vi "2020.1.04生产者消费者地图调用——主vi.vi"() -> ()   [LabVIEW 2018]
uses:
  <vilib>/Instr/_visa.llb/VISA Configure Serial Port (Instr).vi
panel:
  in  "毫秒倍数":u16
  in  "滑动杆":u8(slide) scale=10.0..19.0
  out "十进制合成纬度":dbl format="%#.6g"
  out "十进制合成经度":dbl format="%#.6g"
  out "纬分":dbl
  out "纬度":i32
  out "经分":dbl
  out "经度":i32
  in  "parity (0:none)":enum16{"None", "Odd", "Even", "Mark", "Space"}(ring) caption="奇偶（0:无）"
  in  "data bits (8)":u16=8 caption="数据比特(8)" min=5 max=8 step=1
  in  "baud rate (9600)":u32=9600 caption="波特率(9600)"
  in  "VISA resource name":refnum<visa-resource-name> caption="VISA资源名称"
  in  "WebBrowser":refnum<k7>(container) caption="网页浏览器"
  in  "stop":bool caption="停止"
  out "读取缓冲区":string
  out "定位是否成功":bool
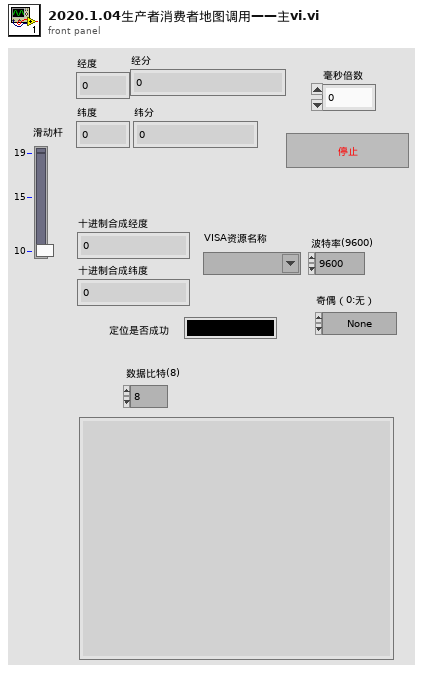
[diagram p1: front panel]
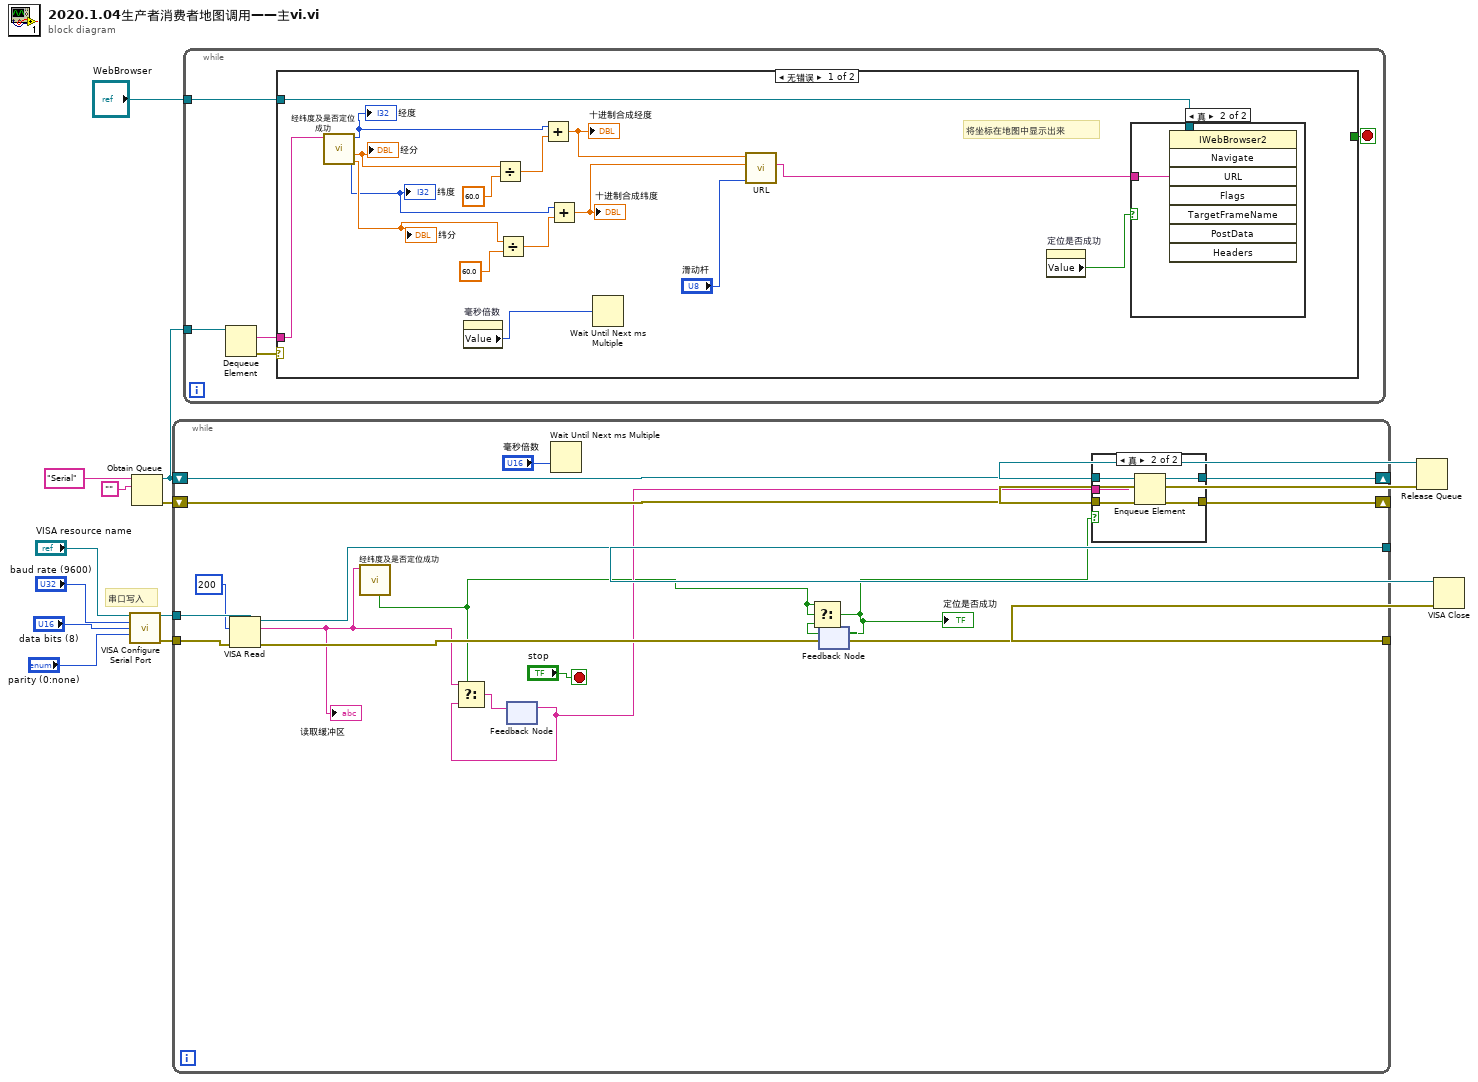
[diagram p0: block diagram]
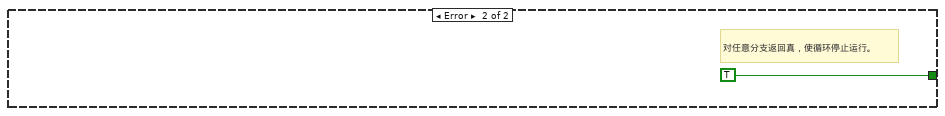
[diagram p3: hidden frame]
diagram:
  # "串口写入"
  n1 = call-poly "VISA Configure Serial Port"("VISA resource name"="VISA resource name", "baud rate (9600)"="baud rate (9600)", "data bits (8)"="data bits (8)", "parity (0:none)"="parity (0:none)") -> ("VISA resource name out"=w12:refnum<visa-resource-name>, "error out"=w10:errorcluster)  [unwired: 10 in]
  n2 = Obtain Queue(name (unnamed)="Serial" ("名称（未命名）"), element data type="") -> (queue out=w8:refnum<queue>, error out=w15:errorcluster)  [unwired: 3 in, 1 out]
  n3 = while {
    shift-right: [w29] -> w13
    shift-left: w15 -> [w28]
    shift-right: [w30] -> w14
    shift-left: w8 -> [w31]
    tunnel: w12 -> [w27]
    tunnel: [w26] -> w11
    tunnel: w10 -> [w24]
    tunnel: [w23] -> w9
    stop <- "stop" stop-if-true
    n4 = VISA Read(VISA resource name=w27, byte count=u32 200 ("字节总数"), error in (no error)=w24) -> (VISA resource name out=w26:refnum<visa-resource-name>, read buffer=w16:string, error out=w23:errorcluster)  [unwired: 1 out]
    "读取缓冲区" <- w16
    n5 = call "经纬度及是否定位成功.vi"("即时数据"=w16) -> ("定位成功"=w20:bool)  [unwired: 6 in, 4 out]
    n6 = feedback #1() -> (w21:string)  [unwired: 1 in]
    n7 = Select(t=w16, s=w20, f=w21) -> (s? t:f=w22:string)
    n8 = feedback-in #1(w22) -> ()
    n9 = Wait Until Next ms Multiple(millisecond multiple="毫秒倍数") -> ()  [unwired: 1 out]
    n10 = feedback #2() -> (w19:bool)  [unwired: 1 in]
    n11 = Select(t=w20, s=w20, f=w19) -> (s? t:f=w18:bool)
    "定位是否成功" <- w18
    n12 = feedback-in #2(w18) -> ()
    n13 = case shown="真" w18 {
      tunnel: w31 -> [w34 w39]
      tunnel: [w34 w38] -> w30
      tunnel: [w33 w36] -> w29
      tunnel: w28 -> [w33 w37]
      tunnel: w21 -> [_ w35]
      frame False {
      }
      frame True {
        n14 = Enqueue Element(queue=w39, element=w35, error in (no error)=w37) -> (queue out=w38:refnum<queue>, error out=w36:errorcluster)  [unwired: 1 in, 1 out]
      }
    }
  }
  n15 = while {
    tunnel: w8 -> [w44]
    tunnel: "WebBrowser" -> [w40]
    stop <- w41 stop-if-true
    n16 = Dequeue Element(queue=w44) -> (element=w42:string, error out=w43:errorcluster)  [unwired: 2 in, 2 out]
    n17 = case shown="无错误" w43 {
      tunnel: w42 -> [w47 _]
      tunnel: [_ TRUE] -> w41
      tunnel: w40 -> [w60 _]
      frame No Error {
        # "将坐标在地图中显示出来"
        n18 = call "经纬度及是否定位成功.vi"("即时数据"=w47) -> ("纬分"=w57:dbl, "纬度"=w53:i32, "经分"=w56:dbl, "经度"=w55:i32)  [unwired: 6 in, 1 out]
        "经度" <- w55
        "经分" <- w56
        "纬度" <- w53
        "纬分" <- w57
        n19 = property on="毫秒倍数" class="DigNum (严格)"() -> ("Value"=w48:u16)  [unwired: 2 in, 2 out]
        n20 = Divide(x=w56, y=60.0) -> (x/y=w54:dbl)
        n21 = Divide(x=w57, y=60.0) -> (x/y=w52:dbl)
        n22 = Add(x=w55, y=w54) -> (x+y=w50:dbl)
        "十进制合成经度" <- w50
        n23 = Add(x=w53, y=w52) -> (x+y=w45:dbl)
        "十进制合成纬度" <- w45
        n24 = Wait Until Next ms Multiple(millisecond multiple=w48) -> ()  [unwired: 1 out]
        n25 = call "URL.vi"("比例尺"="滑动杆", "纬度"=w45, "经度"=w50) -> ("URL"=w49:string)  [unwired: 8 in]
        n26 = property on="定位是否成功" class="Bool (严格)"() -> ("Value"=w51:bool)  [unwired: 2 in, 2 out]
        n27 = case shown="真" w51 {
          tunnel: w60 -> [_ w62]
          tunnel: w49 -> [_ w61]
          frame False {
          }
          frame True {
            n28 = invoke class="IWebBrowser2" method="Navigate"(reference=w62, "URL"=w61) -> ()  [unwired: 6 in, 8 out]
          }
        }
      }
      frame Error {
        # "对任意分支返回真，使循环停止运行。"
      }
    }
  }
  n29 = Release Queue(queue=w14, error in (no error)=w13) -> ()  [unwired: 1 in, 3 out]
  n30 = VISA Close(VISA resource name=w11, error in (no error)=w9) -> ()  [unwired: 1 out]
